vi "CSM - Check If Module Exists.vi"(8 "Error In":errorcluster caption="error in (no error)", 11 "CSM Name":string) -> (0 "error out":errorcluster, 2 "Exist?":bool, 3 "CSM Name (Dup)":string)   [LabVIEW 2017, in "Communicable State Machine.lvlib"]
doc: "### CSM - Check If Module Exists.vi\n\nCheck if the CSM module exists\n\n-- <b>Controls</b> --\n- <b>CSM Name</b>: CSM module name\n\n-- <b>Indicators</b> --\n- <b>Exist?</b>: Returns whether the module exists\n- <b>CSM Name(dup)</b>: Returns <b>CSM Name</b>"
uses:
  Communicable State Machine.lvlib
  _Support/CSMQ/_CSMObj-ModeData.ctl
  _Support/CSMQ/_CSMObj-Data.ctl
  _Support/Priority Queue/Priority Queue.ctl
  _Support/Typedef/_Cross CSM State Data.ctl
  _Support/Typedef/_CSM_MSG_TYPE.ctl
  _Support/Typedef/_Cross CSM State Response.ctl
  _Support/Typedef/_CSM_Response Source Message.ctl
  _Support/Priority Queue/def-Data(LowPRI-Q).ctl
  _Support/CSMQ/_CSMOFGVOPER.ctl
  _Support/ChangeFlag/ChangeFlag-Read.vi
  _Support/ChangeFlag/ChangeFlagDB.vi
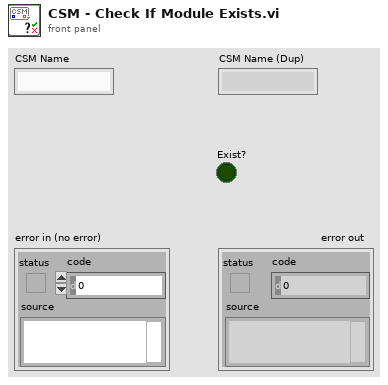
[diagram p1: front panel]
types:
  T1 = typedef "Communicable State Machine.lvlib/_CSMOFGVOPER.ctl" = enum16{"Create If not Exist", "Get By Name", "List", "Check If Name Exists", "Release", "Module Status", "Create Status Event Handler", "Destroy Status Event Handler", "Clear Invalid Objs"}
  T2 = typedef "Communicable State Machine.lvlib/_CSMObj.ctl" = cluster{"info":T3, "Refs":T5}
  T3 = typedef "Communicable State Machine.lvlib/_CSMObj-Info.ctl" = cluster{"Module Name":string, "Requested Name":string, "Group Name":string, "Mode":T4, "Allowed Messages":string[]}
  T4 = typedef "Communicable State Machine.lvlib/_CSM_MODE.ctl" = enum16{"Not Exist", "Stand Alone", "CSM", "Worker", "Worker Agent", "Chain Node", "Chain"}
  T5 = typedef "Communicable State Machine.lvlib/_CSMObj-Refs.ctl" = cluster{"WatchDogQ":refnum<queue>, "CSMDataDVR":refnum<data-value>, "Queue":T6, "GroupDataDVR":refnum<data-value>, "TagMap":refnum<data-value>, "ExitEvent":refnum<user-event>, "NewStateEvent":refnum<user-event>, "StatusChangeEvent":refnum<user-event>}
  T6 = typedef "Communicable State Machine.lvlib/Priority Queue.ctl" = cluster{"HPriorityQ":refnum<queue>, "LowPriorityQ":refnum<queue>}
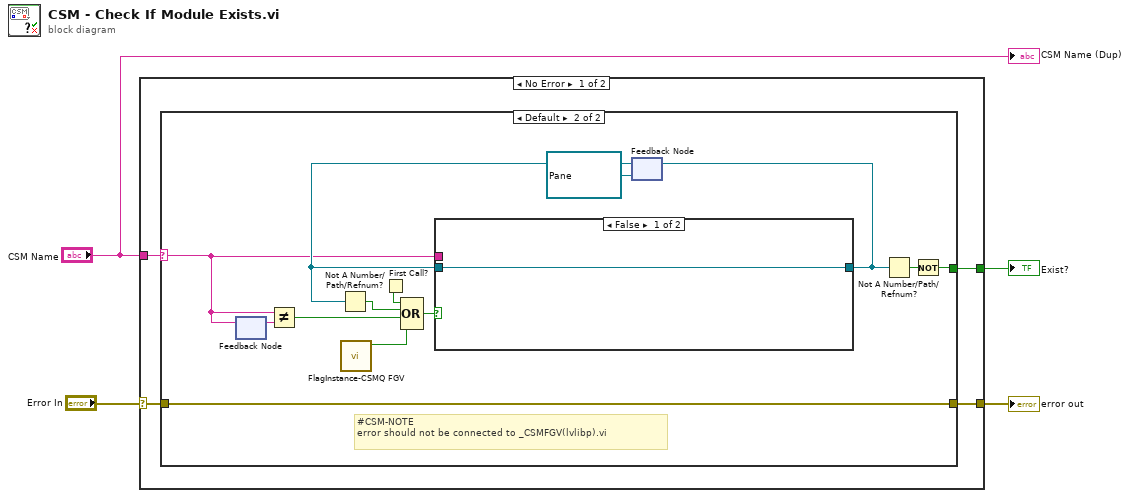
[diagram p0: block diagram]
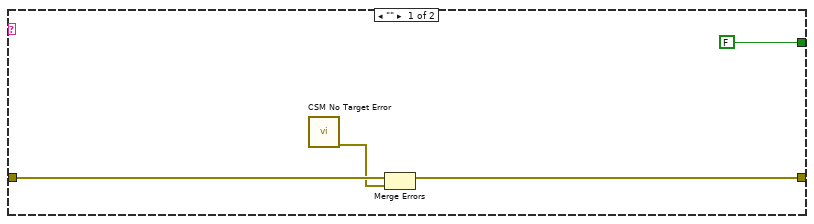
[diagram p2: hidden frame]
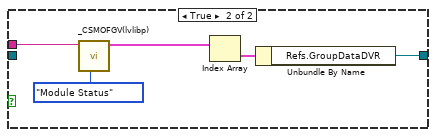
[diagram p3: hidden frame]
diagram:
  n1 = case shown="No Error" "Error In" {
    selector: "Error In" -> [w5 w32]
    tunnel: "CSM Name" -> [w8 _]
    tunnel: [w7 _] -> w3
    tunnel: [w6 w32] -> w1
    frame No Error {
      n2 = case shown="Default" w8 {
        selector: w8 -> [_ w15]
        tunnel: [FALSE w16] -> w7
        tunnel: [w10 w13] -> w6
        tunnel: w5 -> [w11 w13]
        frame "" {
          n3 = call "CSM No Target Error.vi"() -> ("error out"=w9:errorcluster)  [unwired: 11 in]
          n4 = Merge Errors(w11, w9) -> (w10:errorcluster)
        }
        frame Default {
          # "#CSM-NOTE\nerror should not be connected to _CSMFGV(lvlibp).vi"
          n5 = feedback #1() -> (w22:string)  [unwired: 1 in]
          n6 = feedback-in #1(w15) -> ()
          n7 = Not Equal?(x=w15, y=w22) -> (x != y?=w23:bool)
          n8 = call "FlagInstance-CSMQ FGV.vi"() -> ("Changed"=w14:bool)  [unwired: 10 in, 1 out]
          n9 = First Call?() -> (First Call?: T/F=w25:bool)
          n10 = feedback #2(refnum<data-value> refnum ("Mode-Data")) -> (w19:refnum<data-value>)
          n11 = Not A Number/Path/Refnum?(number/path/refnum=w19) -> (NaN/Path/Refnum?=w20:bool)
          n12 = Compound Arithmetic op=OR(w25, w20, w23, w14) -> (w24:bool)
          n13 = case shown="False" w24 {
            tunnel: [w26 w28] -> w17
            tunnel: w19 -> [w26 _]
            tunnel: w15 -> [_ w27]
            frame False {
            }
            frame True {
              n14 = call "_CSMOFGV(lvlibp).vi"("Operation"=_CSMOFGVOPER."Module Status", "Name (\"\" to Use UUID) In"=w27) -> ("Array"=w30:T2[])  [unwired: 7 in, 2 out]
              n15 = Index Array(array=w30) -> (element=w29:T2)  [unwired: 1 in]
              n16 = Unbundle By Name(w29) -> ("Refs.GroupDataDVR"=w28:refnum<data-value>)
            }
          }
          n17 = feedback-in #2(w17) -> ()
          n18 = Not A Number/Path/Refnum?(number/path/refnum=w17) -> (NaN/Path/Refnum?=w18:bool)
          n19 = Not(x=w18) -> (.not. x?=w16:bool)
        }
      }
    }
    frame Error {
    }
  }
  "error out" <- w1
  "Exist?" <- w3
  "CSM Name (Dup)" <- "CSM Name"
